vi "ProdaNG.Configurator.Popup.Release.vi"(9 "Release":bool, 10 "Elements to release/unrelease":T1[](array[typedef])) -> (4 "Reason out":string, 5 "OK?":bool)   [LabVIEW 2016]
uses:
  ProdaNG.Tree.Fglb.Data.ctl
  ProdaNG.Tree.Fglb.Element.ctl
panel:
  in  "Reason":string
  in  "Button.Cancel":bool
  in  "Button.OK":bool
  out "Msg":string
  out "Elements":i32(listbox)
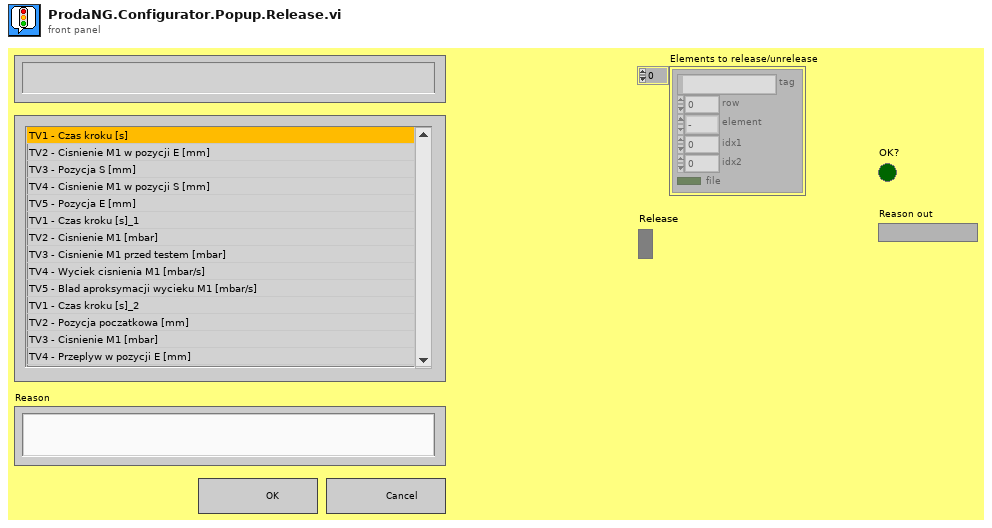
[diagram p1: front panel]
types:
  T1 = typedef "ProdaNG.Tree.Fglb.Data.ctl" = cluster{"tag":string, "row":i32, "element":T2, "idx1":i32, "idx2":i32, "file":bool}
  T2 = typedef "ProdaNG.Tree.Fglb.Element.ctl" = enum16{"-", "PP", "TS", "TP", "TV"}
  T3 = enum8{"Enabled", "Disabled", "Disabled and Grayed Out"}
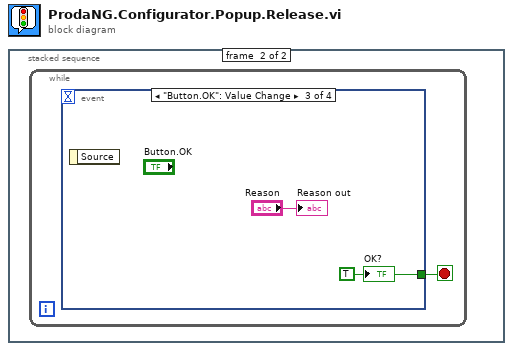
[diagram p0: block diagram]
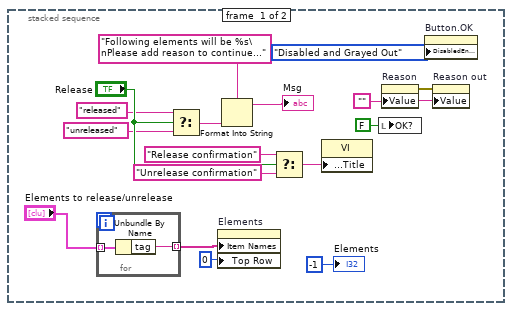
[diagram p2: hidden frame]
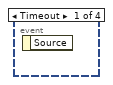
[diagram p3: hidden frame]
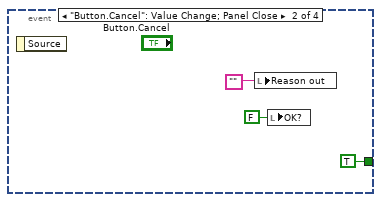
[diagram p4: hidden frame]
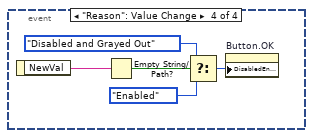
[diagram p5: hidden frame]
diagram:
  n1 = stacked-sequence {
    frame #0 {
      w1 = ""
      n2 = for {
        tunnel: "Elements to release/unrelease" -> [w19] mode=indexing
        tunnel: [w18] -> w5 mode=indexing
        n3 = Unbundle By Name(w19) -> ("tag"=w18:string)
      }
      n4 = Select(t="released" ("Front Panel Window:Title"), s="Release", f="unreleased" ("Front Panel Window:Title")) -> (s? t:f=w9:string)
      n5 = property on="Elements" class="LstBox (strict)"("Item Names"=w5, "Top Row"=0) -> ()  [unwired: 2 in, 2 out]
      n6 = Format Into String(format string="Following elements will be %s\nPlease add reason to continue..." ("Msg"), w9) -> (resulting string=→"Msg":string)  [unwired: 2 in, 1 out]
      n7 = Select(t="Release confirmation" ("Front Panel Window:Title"), s="Release", f="Unrelease confirmation" ("Front Panel Window:Title")) -> (s? t:f=w15:string)
      n8 = property class="VI"("Front Panel.Title"=w15) -> ()  [unwired: 2 in, 2 out]
      n9 = local write "OK?"(FALSE ("OK?")) -> ()
      n10 = property on="Reason" class="Str"("Value"=w1) -> (error out=w2:errorcluster)  [unwired: 2 in, 1 out]
      n11 = property on="Button.OK" class="Bool"("DisabledEnum"=T3."Disabled and Grayed Out" ("Disabled")) -> ()  [unwired: 2 in, 2 out]
      n12 = property on="Reason out" class="Str"(error in=w2, "Value"=w1) -> ()  [unwired: 1 in, 2 out]
      "Elements" <- -1 ("Elements")
    }
    frame #1 {
      n13 = while {
        stop <- w20 stop-if-true
        n14 = event shown="[2] \"Button.OK\": Value Change" {
          selector: _ -> [_ _ _ _]
          dyn-events: _ -> [_ _ _ _]
          timeout: _ -> [_ _ _ _]
          tunnel: [_ TRUE ("OK?") w25 _] -> w20
          event Timeout {
            n15 = event-data() -> ()  [unwired: 1 in, 1 out]
          }
          event "Button.Cancel": Value Change; Panel Close {
            n16 = event-data() -> ()  [unwired: 1 in, 1 out]
            n17 = local write "Reason out"("") -> ()
            n18 = local write "OK?"(FALSE ("OK?")) -> ()
          }
          event "Button.OK": Value Change {
            w25 = TRUE ("OK?")
            n19 = event-data() -> ()  [unwired: 1 in, 1 out]
            "OK?" <- w25
            "Reason out" <- "Reason"
          }
          event "Reason": Value Change {
            n20 = event-data() -> ("NewVal"=w30:string)  [unwired: 1 in]
            n21 = Empty String/Path?(string/path=w30) -> (empty?=w29:bool)
            n22 = Select(t=T3."Disabled and Grayed Out" ("Disabled"), s=w29, f=T3."Enabled" ("Disabled")) -> (s? t:f=w26:T3)
            n23 = property on="Button.OK" class="Bool"("DisabledEnum"=w26) -> ()  [unwired: 2 in, 2 out]
          }
        }
      }
    }
  }
